vi "Close Line Followers.vi"(8 "error in":errorcluster) -> (0 "error out":errorcluster)   [LabVIEW 2018]
uses:
  TypeDefs/typedef_enum_Refnums.ctl
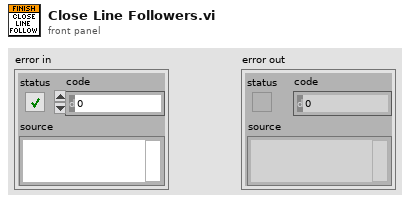
[diagram p1: front panel]
types:
  T1 = typedef "typedef_enum_Refnums.ctl" = enum16{"Ball_Encoder", "Ball_Motor", "Camera", "Linefollow_3", "Linefollow_2", "Linefollow_1", "Gyro", "Hatch_Solenoid", "Climb_Back_Solenoid", "Arm_Encoder", "Arm_Motor", "Lift_Encoder", "Drive", "Drive_Motor_R", "Drive_Motor_L", "Drive_Encoder_R", "Drive_Encoder_L", "Joy_R", "Joy_L", "Wrist_Motor", "Wrist_Encoder", "Climb Upper Limit", "Climb Lower Limit ", "Climb_Front_Motor"}
  T2 = typedef "WPI_DigitalInputDevRef.ctl" = cluster{"DevStatus":errorcluster, "DIO Channel":T3}
  T3 = typedef "FPGA_DIOChannel.ctl" = enum8{"DIO 0", "DIO 1", "DIO 2", "DIO 3", "DIO 4", "DIO 5", "DIO 6", "DIO 7", "DIO 8", "DIO 9", "DIO MXP 0", "DIO MXP 1", "DIO MXP 2", "DIO MXP 3", "DIO MXP 4", "DIO MXP 5", "DIO MXP 6", "DIO MXP 7", "DIO MXP 8", "DIO MXP 9", "DIO MXP 10", "DIO MXP 11", "DIO MXP 12", "DIO MXP 13", "DIO MXP 14", "DIO MXP 15", "SPI Port CS1", "SPI Port CS2", "SPI Port CS3", "SPI Port MISO", "SPI Port MOSI", "Invalid"}
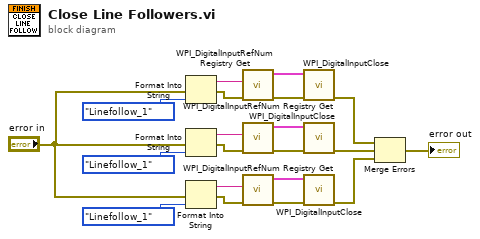
[diagram p0: block diagram]
diagram:
  n1 = Format Into String(error in="error in", typedef_enum_Refnums."Linefollow_1" ("RefNums")) -> (resulting string=w18:string, error out=w17:errorcluster)  [unwired: 2 in]
  n2 = Format Into String(error in="error in", typedef_enum_Refnums."Linefollow_1" ("RefNums")) -> (resulting string=w13:string, error out=w14:errorcluster)  [unwired: 2 in]
  n3 = Format Into String(error in="error in", typedef_enum_Refnums."Linefollow_1" ("RefNums")) -> (resulting string=w8:string, error out=w7:errorcluster)  [unwired: 2 in]
  n4 = call <vilib>:"WPI_DigitalInputRefNum Registry Get.vi"("error in (no error)"=w17, "refnum name"=w18) -> ("error out"=w20:errorcluster, "DigitalInputDevRef"=w19:T2)  [unwired: 8 in]
  n5 = call <vilib>:"WPI_DigitalInputRefNum Registry Get.vi"("error in (no error)"=w14, "refnum name"=w13) -> ("error out"=w11:errorcluster, "DigitalInputDevRef"=w12:T2)  [unwired: 8 in]
  n6 = call <vilib>:"WPI_DigitalInputRefNum Registry Get.vi"("error in (no error)"=w7, "refnum name"=w8) -> ("error out"=w10:errorcluster, "DigitalInputDevRef"=w9:T2)  [unwired: 8 in]
  n7 = call <vilib>:"WPI_DigitalInputClose.vi"("error in (no error)"=w20, "DigitalInputDevRef"=w19) -> ("error out"=w4:errorcluster)  [unwired: 9 in]
  n8 = call <vilib>:"WPI_DigitalInputClose.vi"("error in (no error)"=w11, "DigitalInputDevRef"=w12) -> ("error out"=w3:errorcluster)  [unwired: 9 in]
  n9 = call <vilib>:"WPI_DigitalInputClose.vi"("error in (no error)"=w10, "DigitalInputDevRef"=w9) -> ("error out"=w2:errorcluster)  [unwired: 9 in]
  n10 = Merge Errors(w4, w3, w2) -> (→"error out":errorcluster)
